vi "Write to File.vi"(8 "error in":errorcluster, 11 "xData in":refnum<class "xData.lvclass">) -> (0 "error out":errorcluster, 2 "Serialized Data Out":string, 3 "xData out":refnum<class "xData.lvclass">)   [LabVIEW 2014, in "xData.lvclass"]
uses:
  xData.lvclass
  PAS/Data/Cell/ePAS Cell Data.lvclass
  reusable/CRDS/Data/Cell/CRDS Cell Data.lvclass
  reusable/PAS/Data/Main/PAS Data.lvclass
  reusable/CRDS/Data/Main/CRDS Data.lvclass
  reusable/CRDS/Cell/extParam Ctl.ctl
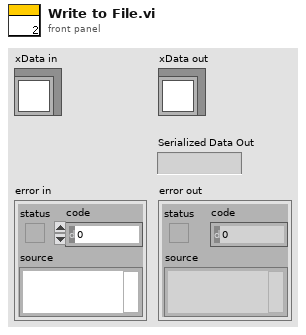
[diagram p1: front panel]
types:
  T1 = typedef "CRDS Lib.lvlib/CRDS Cell Data.lvclass/extParam Ctl.ctl" = cluster{"Tau":sgl, "Tau0cor":sgl, "ext":sgl, "extCorr":sgl, "stdevTau":sgl, "eTau":sgl, "taucorr":sgl, "Tau0":sgl, "max":sgl}
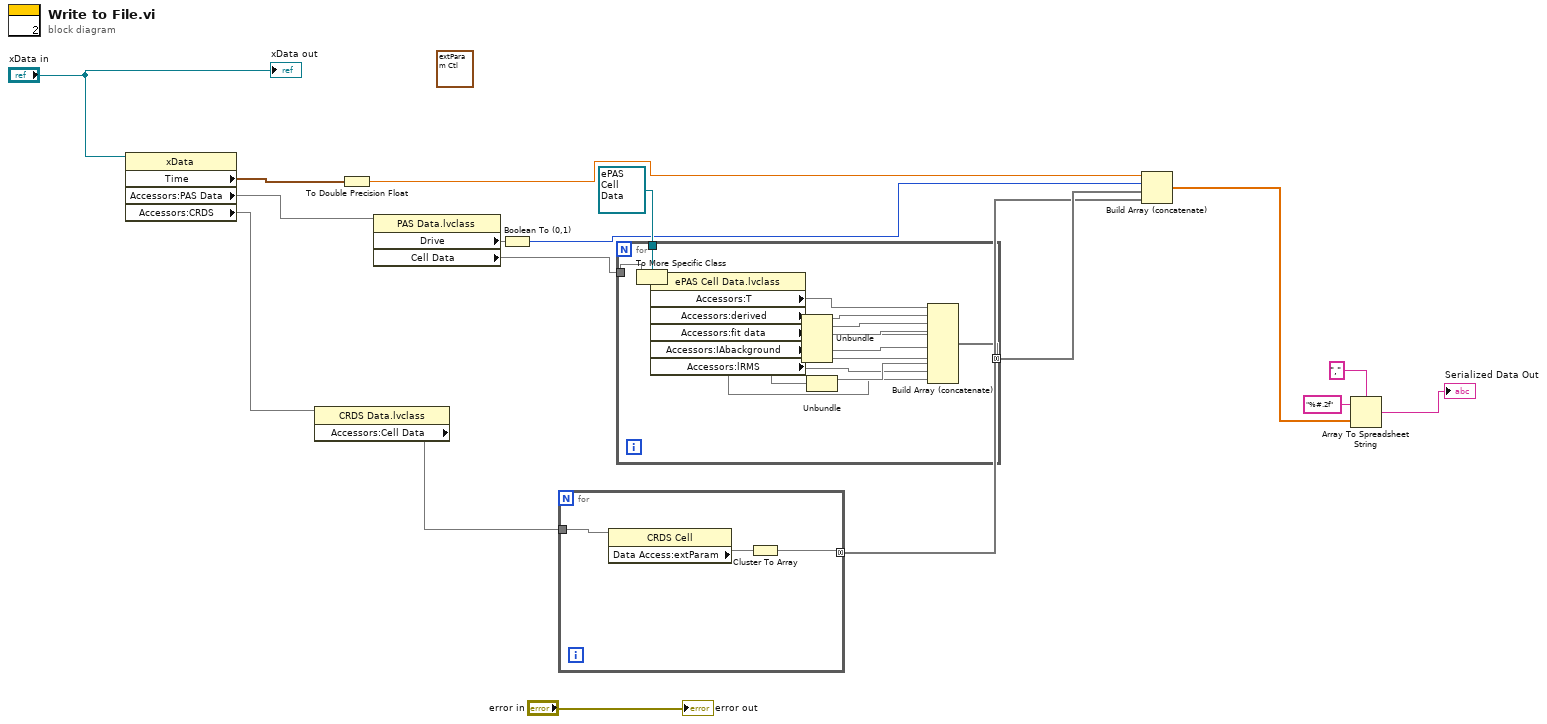
[diagram p0: block diagram]
diagram:
  (unwired) T1 {"Tau"=nan, "Tau0cor"=nan, "ext"=nan, "extCorr"=nan, "stdevTau"=nan, "eTau"=nan, "taucorr"=nan, "Tau0"=nan, "max"=nan} ("extParam")
  n1 = property class="xData"(reference="xData in") -> ("Time"=w15:timestamp, "Accessors:PAS Data"=w14, "Accessors:CRDS"=w7)  [unwired: 1 in, 2 out]
  n2 = property class="CRDS Data.lvclass"(reference=w7) -> ("Accessors:Cell Data"=w6)  [unwired: 1 in, 2 out]
  n3 = To Double Precision Float(number=w15) -> (double precision float=w11:dbl)
  n4 = property class="PAS Data.lvclass"(reference=w14) -> ("Drive"=w8, "Cell Data"=w13)  [unwired: 1 in, 2 out]
  n5 = Boolean To (0,1)(Boolean=w8) -> (0, 1=w10:i16)
  n6 = for {
    tunnel: w6 -> [w20]
    tunnel: [w18] -> w5 mode=concatenating
    n7 = property class="CRDS Cell"(reference=w20) -> ("Data Access:extParam"=w19)  [unwired: 1 in, 2 out]
    n8 = Cluster To Array(cluster=w19) -> (array=w18:void[])
  }
  n9 = for {
    tunnel: w13 -> [w37]
    tunnel: refnum<class "ePAS Cell Data.lvclass"> refnum ("ePAS Cell") -> [w36]
    tunnel: [w21] -> w9 mode=concatenating
    n10 = To More Specific Class(target class=w36, reference=w37) -> (specific class reference=w35:refnum<class "ePAS Cell Data.lvclass">, error out=w34:errorcluster)  [unwired: 1 in]
    n11 = property class="ePAS Cell Data.lvclass"(reference=w35, error in=w34) -> ("Accessors:T"=w33, "Accessors:derived"=w32, "Accessors:fit data"=w25, "Accessors:IAbackground"=w23, "Accessors:lRMS"=w22)  [unwired: 2 out]
    n12 = Unbundle(w32) -> (w31, w30, w29, w28, w27, w26)
    n13 = Unbundle(w25) -> (w24)  [unwired: 1 out]
    n14 = Build Array (concatenate)(w33, w31, w30, w29, w28, w27, w26, w24, w23, w22) -> (w21:void[])
  }
  n15 = Build Array (concatenate)(w11, w10, w9, w5) -> (w4:dbl[])
  n16 = Array To Spreadsheet String(delimiter (Tab)=",", array=w4, 3:"%#.2f" ("format string")) -> (spreadsheet string=→"Serialized Data Out":string)
  "error out" <- "error in"
  "xData out" <- "xData in"
